vi "Load Image From File.vi"   [LabVIEW 2020, in "G-Image.lvlib"]
doc: "<b>This VI is polymorphic.</b>\n\nLoad an image file from disk, and return it as a LabVIEW picture.\n\n<b>Path In</b> can be a standard path type, or a UTF-8 encoded string."
uses:
  G-Image.lvlib
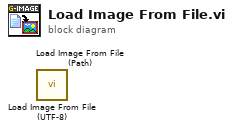
[diagram p0: block diagram]
diagram:
  n1 = call "Load Image From File (UTF-8).vi"() -> ()  [unwired: 9 in, 3 out]
  n2 = call "Load Image From File (Path).vi"() -> ()  [unwired: 9 in, 3 out]
